vi "3.11-Shallow History Map.vi"() -> ()   [LabVIEW 2010]
uses:
  4-High Neurons/4.0-Timing Badass.ctl
  3.0-Global.vi
  <vilib>/Analysis/Matrix/Numeric/Conversions/Matrix To Array - RM.vi
  <vilib>/Analysis/Matrix/Numeric/Conversions/Array To Matrix - RA2.vi
  <vilib>/Analysis/baseanly.llb/Real A x B.vi
  <vilib>/Analysis/Matrix/NI_Matrix.lvlib
  <vilib>/Analysis/NI_AALBase.lvlib
panel:
  out "Local Map time":T1
  in  "Magnitude Array":dbl[](array[numeric])
  in  "Angle Array":dbl[](array[numeric])
  out "XY Graph":cluster{"Y":dbl, "X":dbl}[](graph)
  in  "Current Heading":dbl
  in  "Move Threshold (mm)":i32=100
  in  "Rob Pos Y (mm)":dbl
  in  "Rob Pos X (mm)":dbl
  in  "Distance to Back Axel (mm)":i32=840
  out "Y (mm)":dbl[](array[numeric])
  out "X (mm)":dbl[](array[numeric])
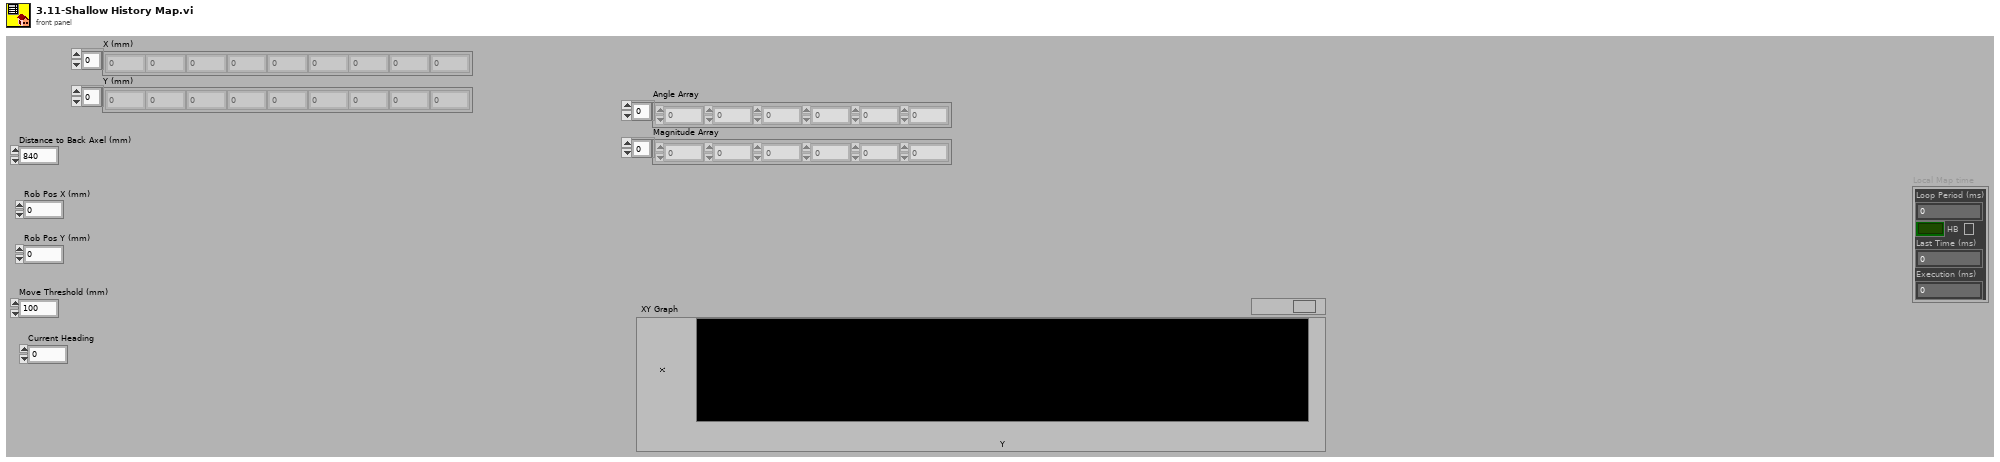
[diagram p1: front panel]
types:
  T1 = typedef "4.0-Timing Badass.ctl" = cluster{"Loop Period (ms)":u32, "HB":bool, "Last Time (ms)":u32, "Execution (ms)":u32}
  T2 = typedef "NI_Matrix.lvlib/RealMatrix.ctl" = dbl[][]
  T3 = cluster{" Angle":dbl, " Magnitude":dbl, " Start Turn":dbl, "X":dbl, "Y":dbl}[]
  T4 = cluster{"Angle":dbl, "Magnitude":dbl, " Start Turn":dbl, "X":dbl, "Y":dbl}[]
  T5 = cluster{"Angle":dbl, "Magnitude":dbl, " Start Turn":dbl, "X":dbl, "Y":dbl}
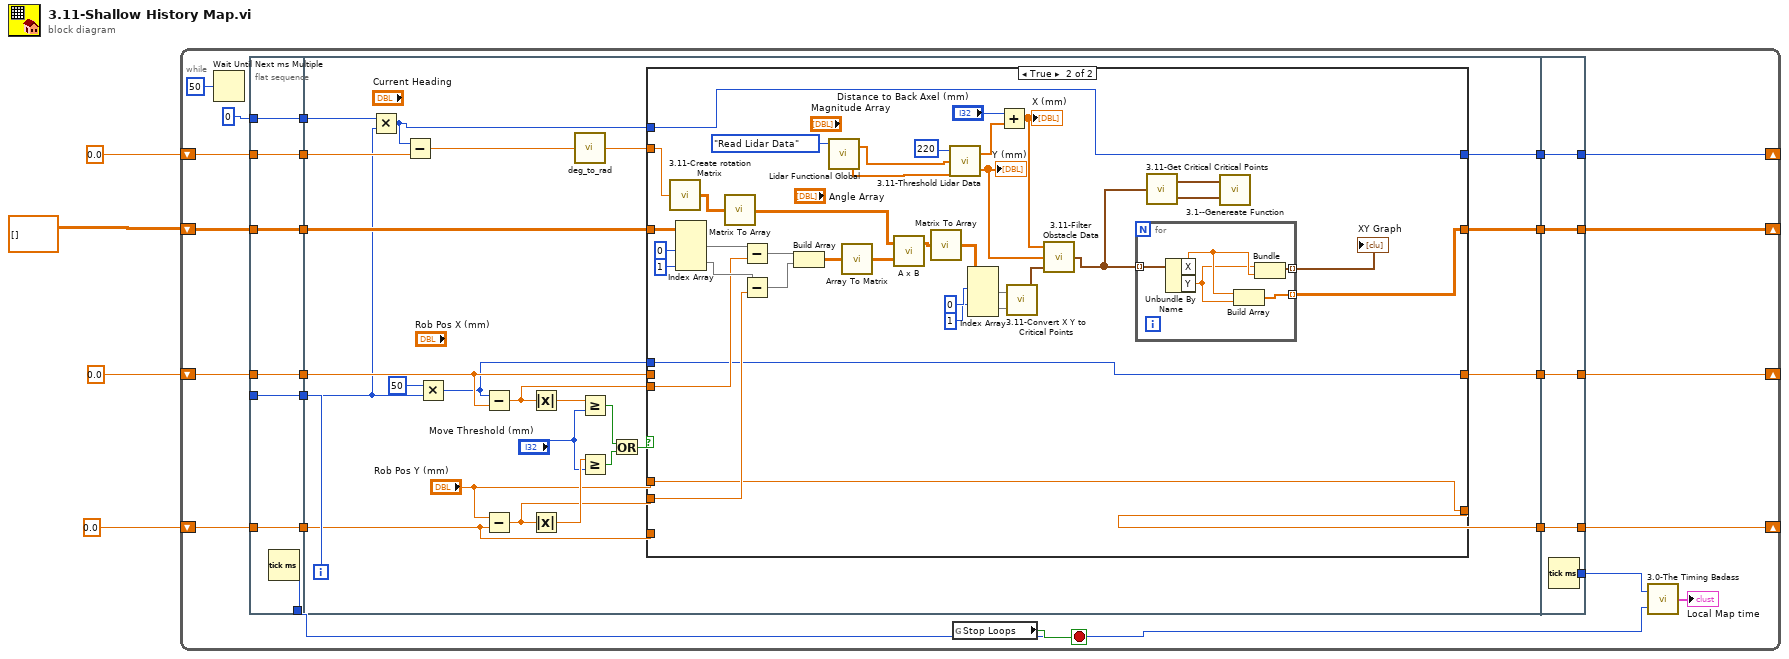
[diagram p0: block diagram]
diagram:
  n1 = while {
    shift-right: [w24] -> _
    shift-left: dbl[][] [] -> [w25]
    shift-right: [w27] -> _
    shift-left: 0.0 -> [w29]
    shift-right: [w26] -> _
    shift-left: 0.0 -> [w28]
    shift-right: [w23] -> _
    shift-left: 0.0 -> [w20]
    i -> [w19]
    stop <- w22 stop-if-true
    n2 = Wait Until Next ms Multiple(millisecond multiple=u32 50) -> ()  [unwired: 1 out]
    n3 = flat-sequence {
      tunnel: w19 -> [w31]
      tunnel: w20 -> [w32]
      tunnel: 0 ("x") -> [w33]
      tunnel: w25 -> [w34]
      tunnel: w28 -> [w35]
      tunnel: w29 -> [w36]
      tunnel: [w36] -> w18
      tunnel: [w35] -> w17
      tunnel: [w34] -> w16
      tunnel: [w33] -> w15
      tunnel: [w32] -> w14
      tunnel: [w31] -> w13
      tunnel: [w30] -> w6
      tunnel: w18 -> [w54]
      tunnel: w17 -> [w53]
      tunnel: w16 -> [w50]
      tunnel: w15 -> [w40]
      tunnel: w14 -> [w39]
      tunnel: w13 -> [w37]
      tunnel: [w52] -> w12
      tunnel: [w51] -> w11
      tunnel: [w47] -> w10
      tunnel: [w46] -> w9
      tunnel: [w108] -> w23
      tunnel: [w109] -> w24
      tunnel: [w110] -> w26
      tunnel: [w111] -> w27
      tunnel: w12 -> [w111]
      tunnel: w11 -> [w110]
      tunnel: w10 -> [w109]
      tunnel: w9 -> [w108]
      tunnel: [w107] -> w7
      frame #0 {
        n4 = Tick Count (ms)() -> (millisecond timer value=w30:u32)
      }
      frame #1 {
        n5 = Multiply(x=w40, y=w37) -> (x*y=w38:i32)
        n6 = Subtract(x=w38, y=w39) -> (x-y=w45:dbl)
        n7 = Multiply(x=50, y=w37) -> (x*y=w42:i32)
        n8 = Subtract(x=w42, y=w54) -> (x-y=w49:dbl)
        n9 = Subtract(x="Rob Pos Y (mm)", y=w53) -> (x-y=w48:dbl)
        n10 = Absolute Value(x=w49) -> (abs(x)=w60:dbl)
        n11 = Absolute Value(x=w48) -> (abs(x)=w59:dbl)
        n12 = call "deg_to_rad.vi"("Degrees"=w45) -> ("Radians"=w44:dbl)
        n13 = Greater Or Equal?(x=w60, y="Move Threshold (mm)") -> (x >= y?=w55:bool)
        n14 = Greater Or Equal?(x=w59, y="Move Threshold (mm)") -> (x >= y?=w56:bool)
        n15 = Or(x=w55, y=w56) -> (x .or. y?=w57:bool)
        n16 = case shown="True" w57 {
          tunnel: w54 -> [w64 _]
          tunnel: w53 -> [w63 _]
          tunnel: [w64 w80] -> w52
          tunnel: [w63 w81] -> w51
          tunnel: w42 -> [_ w80]
          tunnel: "Rob Pos Y (mm)" -> [_ w81]
          tunnel: w50 -> [w62 w98]
          tunnel: w49 -> [_ w94]
          tunnel: w48 -> [_ w95]
          tunnel: [w62 w76] -> w47
          tunnel: [w61 w82] -> w46
          tunnel: w38 -> [w61 w82]
          tunnel: w44 -> [_ w86]
          frame False {
          }
          frame True {
            n17 = call "3.11-Create rotation Matrix.vi"("Radians"=w86) -> ("appended array"=w84:dbl[][])
            n18 = Index Array(array=w98, index (col) #1=0 ("disabled index (col)"), index (col) #2=1 ("index (col)")) -> (element #1=w97:dbl[], element #2=w96:dbl[])  [unwired: 2 in]
            n19 = call-poly <vilib>:"Matrix To Array.vi"("Real Matrix"=w84) -> ("Real 2D Array"=w85:dbl[][])
            n20 = Subtract(x=w97, y=w94) -> (x-y=w93:dbl[])
            n21 = Subtract(x=w96, y=w95) -> (x-y=w92:dbl[])
            n22 = Build Array(w93, w92) -> (w91:dbl[][])
            n23 = call "Lidar Functional Global.vi"("Lidar Action"=enum16{"Set Lidar Data", "Read Lidar Data"}."Read Lidar Data") -> ("Lidar Angle Data Out (Degrees)"=w65:sgl[], "Lidar Magnitude Data Out (mm)"=w66:sgl[])  [unwired: 2 in]
            n24 = call-poly <vilib>:"Array To Matrix.vi"("Real 2D Array"=w91) -> ("Real Matrix"=w88:T2)
            n25 = call-poly <vilib>:"A x B.vi"("B"=w88, "A"=w85) -> ("A x B"=w87:T2)  [unwired: 1 out]
            n26 = call-poly <vilib>:"Matrix To Array.vi"("Real Matrix"=w87) -> ("Real 2D Array"=w75:dbl[][])
            n27 = call "3.11-Threshold Lidar Data.vi"("Angle Array"=w65, "Magnitude Array"=w66, "Local Map Threshold (mm)"=220) -> ("Y (mm)"=w78:dbl[], "X (mm)"=w100:dbl[])
            "Y (mm)" <- w78
            n28 = Index Array(array=w75, index (row) #1=0 ("disabled index (col)"), index (row) #2=1 ("index (col)")) -> (element #1=w74:dbl[], element #2=w73:dbl[])  [unwired: 2 in]
            n29 = Add(x="Distance to Back Axel (mm)", y=w100) -> (x+y=w79:dbl[])
            "X (mm)" <- w79
            n30 = call "3.11-Convert X Y to Critical Points.vi"("Y (mm)"=w73, "X (mm)"=w74) -> ("Array"=w72:T3)
            n31 = call "3.11-Filter Obstacle Data.vi"("Obstacle Array"=w72, "Y Array"=w78, "X Array"=w79) -> ("output array"=w69:T4)
            n32 = for {
              tunnel: w69 -> [w105] mode=indexing
              tunnel: [w106] -> w77 mode=indexing
              tunnel: [w104] -> w76 mode=indexing
              n33 = Unbundle By Name(w105) -> ("X"=w103:dbl, "Y"=w102:dbl)
              n34 = Build Array(w103, w102) -> (w104:dbl[])
              n35 = Bundle("Y"=w102, "X"=w103) -> (w106:cluster{"Y":dbl, "X":dbl})  [unwired: 1 in]
            }
            "XY Graph" <- w77
            n36 = call "3.11-Get Critical Critical Points.vi"("Critical Points"=w69) -> ("Left Data"=w67:T5, "Right Data"=w68:T5)
            n37 = call "3.1--Genereate Function.vi"("Left Data"=w67, "Right Data"=w68) -> ()  [unwired: 1 out]
          }
        }
      }
      frame #2 {
        n38 = Tick Count (ms)() -> (millisecond timer value=w107:u32)
      }
    }
    n39 = global read "3.0-Global.vi" "Stop Loops"() -> (w22:bool)
    n40 = call "3.0-The Timing Badass.vi"("Start"=w6, "End"=w7) -> ("Super Heart Beat"=→"Local Map time":T1)
  }
